vi "FeedForward.vi"(9 "opinons":dbl[](array[numeric]), 10 "inputs":dbl[][](array[numeric])) -> (2 "output":dbl[](array[numeric]))   [LabVIEW 2014]
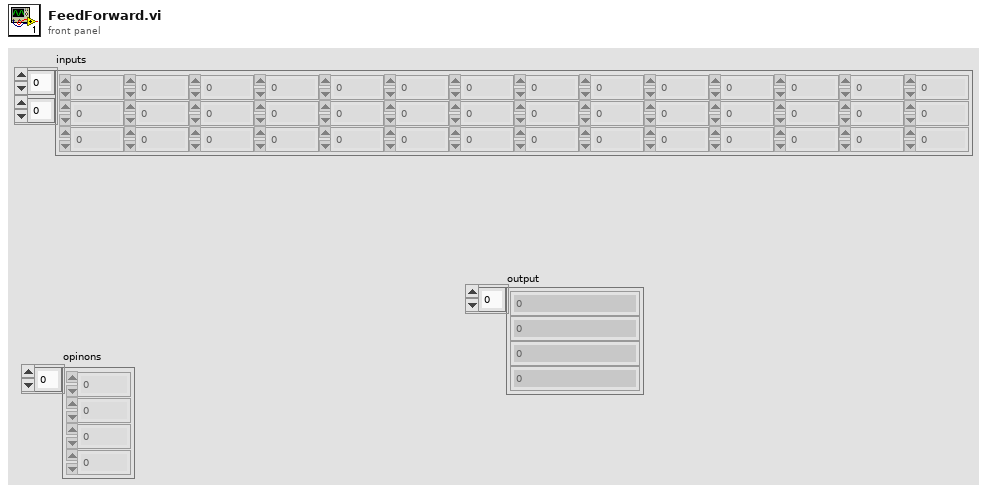
[diagram p1: front panel]
types:
  T1 = enum16{"Single Node", "1 Hidden Level", "2 Hidden Levels"}
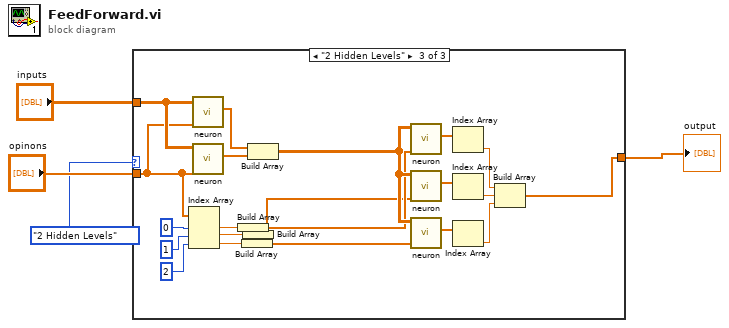
[diagram p0: block diagram]
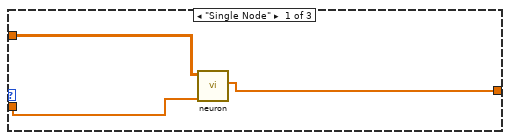
[diagram p2: hidden frame]
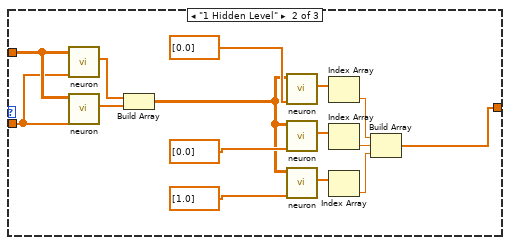
[diagram p3: hidden frame]
diagram:
  n1 = case shown="\"2 Hidden Levels\"" T1."2 Hidden Levels" {
    tunnel: [w5 w9 w33] -> w4
    tunnel: "inputs" -> [w7 w21 w42]
    tunnel: "opinons" -> [w6 w8 w29]
    frame "Single Node" {
      n2 = call "neuron.vi"("opinons"=w6, "inputs"=w7) -> ("output"=w5:dbl[])  [unwired: 9 in]
    }
    frame "1 Hidden Level" {
      n3 = call "neuron.vi"("opinons"=w8, "inputs"=w21) -> ("output"=w20:dbl[])  [unwired: 9 in]
      n4 = call "neuron.vi"("opinons"=w8, "inputs"=w21) -> ("output"=w22:dbl[])  [unwired: 9 in]
      n5 = Build Array(w20, w22) -> (w16:dbl[][])
      n6 = call "neuron.vi"("opinons"=dbl[] [0.0], "inputs"=w16) -> ("output"=w15:dbl[])  [unwired: 9 in]
      n7 = call "neuron.vi"("opinons"=dbl[] [0.0], "inputs"=w16) -> ("output"=w14:dbl[])  [unwired: 9 in]
      n8 = call "neuron.vi"("opinons"=dbl[] [1.0], "inputs"=w16) -> ("output"=w13:dbl[])  [unwired: 9 in]
      n9 = Index Array(array=w15) -> (element=w10:dbl)  [unwired: 1 in]
      n10 = Index Array(array=w14) -> (element=w11:dbl)  [unwired: 1 in]
      n11 = Index Array(array=w13) -> (element=w12:dbl)  [unwired: 1 in]
      n12 = Build Array(w10, w11, w12) -> (w9:dbl[])
    }
    frame "2 Hidden Levels" {
      n13 = Index Array(array=w29, index #1=0 ("index"), index #2=1 ("index"), index #3=2 ("index")) -> (element #1=w28:dbl, element #2=w26:dbl, element #3=w27:dbl)
      n14 = call "neuron.vi"("opinons"=w29, "inputs"=w42) -> ("output"=w41:dbl[])  [unwired: 9 in]
      n15 = call "neuron.vi"("opinons"=w29, "inputs"=w42) -> ("output"=w43:dbl[])  [unwired: 9 in]
      n16 = Build Array(w28) -> (w25:dbl[])
      n17 = Build Array(w27) -> (w23:dbl[])
      n18 = Build Array(w26) -> (w24:dbl[])
      n19 = Build Array(w41, w43) -> (w40:dbl[][])
      n20 = call "neuron.vi"("opinons"=w25, "inputs"=w40) -> ("output"=w39:dbl[])  [unwired: 9 in]
      n21 = call "neuron.vi"("opinons"=w24, "inputs"=w40) -> ("output"=w38:dbl[])  [unwired: 9 in]
      n22 = call "neuron.vi"("opinons"=w23, "inputs"=w40) -> ("output"=w37:dbl[])  [unwired: 9 in]
      n23 = Index Array(array=w39) -> (element=w34:dbl)  [unwired: 1 in]
      n24 = Index Array(array=w38) -> (element=w35:dbl)  [unwired: 1 in]
      n25 = Index Array(array=w37) -> (element=w36:dbl)  [unwired: 1 in]
      n26 = Build Array(w34, w35, w36) -> (w33:dbl[])
    }
  }
  "output" <- w4
